vi "HOST_feedbacktest1_AAoptAOD_8-8-23.vi"() -> ()   [LabVIEW 2020]
uses:
  <vilib>/userDefined/Silver/nirio_resource_slv.ctl
  Controls/Clock Select.ctl
  <vilib>/rvi/Analysis/control/PID/Typedef/niFpgaPID_ManualControl.ctl
  <vilib>/rvi/Analysis/control/PID/Typedef/niFpgaPID_PIDGains.ctl
  <vilib>/rvi/Analysis/control/PID/Typedef/niFpgaPID_OutputRange.ctl
  <vilib>/rvi/Analysis/control/PID/Typedef/niFpgaPID_SetpointWeightings.ctl
  <vilib>/rvi/Analysis/host/Butterworth/config/Butterworth Filter Order.ctl
  <vilib>/rvi/Analysis/host/Butterworth/config/Butterworth Filter Type.ctl
  <vilib>/FPGAPlugInAG/PXIe-7972R/niLvFpga_Open_PXIe-7972R.vi
  <vilib>/rvi/interface/common/dynamic/niFpgaDynamicAddResources.vi
  <vilib>/rvi/interface/common/niFpgaWaitOnOcc.vi
  <vilib>/Utility/error.llb/Error Cluster From Error Code.vi
  <vilib>/rvi/Analysis/host/Butterworth/config/BwScaledCoefficients.vi
  <vilib>/Utility/file.llb/Write Delimited Spreadsheet (string).vi
  <vilib>/rvi/errors/niLvFpgaAdjustHostInterfaceError.vi
  <instrlib>/_niInstr/Streaming/v1/Host/Public/Start Finite Stream.vi
  <instrlib>/_niInstr/Streaming/v1/Host/Public/Wait for Stream.vi
  <instrlib>/_niInstr/Streaming/v1/Host/Public/Start Continuous Stream.vi
  <vilib>/FPGAPlugInAG/Dynamic/niLvFpga_Close_Dynamic.vi
  <vilib>/rvi/interface/nirviOpenFPGA/nirviOpenFPGA.xnode
  FPGA Bitfiles/rfsignal_FPGATarget_feedbacktest1AAo_8pa4StVbrw0.lvbitx
  <vilib>/rvi/interface/nirviMethod/nirviMethod.xnode
  <vilib>/rvi/Analysis/host/Butterworth/XNode/ButterworthCoefficients.xnode
  <vilib>/rvi/interface/nirviReadWriteControl/nirviReadWriteControl.xnode
  <vilib>/rvi/interface/nirviCloseFPGA/nirviCloseFPGA.xnode
  <vilib>/rvi/errors/niLvFpgaMergeErrorWithErrorCode.vi
  <instrlib>/_niInstr/Streaming/v1/Host/niInstr Streaming v1 Host.lvlib
  <vilib>/rvi/interface/Simulation/niFpgaSimulationCallBeginRW.vi
  NiFpgaLv.dll
  <vilib>/rvi/Analysis/host/Public/NI_FpgaMspHost.lvlib
  <vilib>/FPGAPlugInAG/Dynamic/niLvFpga_ConfigureFifo_Dynamic.vi
  <vilib>/FPGAPlugInAG/Dynamic/niLvFpga_StartFifo_Dynamic.vi
  <vilib>/FPGAPlugInAG/Dynamic/niLvFpga_WriteFifo_Dynamic.vi
panel:
  in  "hp freq X 1":dbl=1300.0
  in  "lp freq X 1":dbl=1300.0
  in  "Setpoint Y 2":i16
  in  "Lower lim Y 2":fxp<+/-,16,16>=-300.0
  in  "Upper lim Y 2":fxp<+/-,16,16>=300.0
  in  "D (Y)2":fxp<+/-,16,16>
  in  "I (X)":fxp<+/-,16,16>
  in  "P (X)":fxp<+/-,16,16>
  in  "setpoint weighting 2":T1={"proportional weighting (1)"=1.0, "derivative weighting (0)"=0.0} {"derivative weighting (0)" min=0 max=1; "proportional weighting (1)" min=0 max=1}
  in  "output range 2":T2={"output high (Inf)"=inf, "output low (-Inf)"=-inf}
  in  "gains 2":T3 {"filter coefficient" min=0 max=1; "proportional gain" step=0.125}
  in  "manual control 2":T4
  in  "channel (0) 2":u8
  in  "reset? (F) 2":bool
  in  "Direction switch":bool
  in  "Step gain values":dbl
  in  "?":bool
  in  "% of max CH 1":dbl=85.0
  in  "% of max CH 0":dbl=85.0
  in  "setpoint weighting":T1={"proportional weighting (1)"=1.0, "derivative weighting (0)"=0.0} {"derivative weighting (0)" min=0 max=1; "proportional weighting (1)" min=0 max=1}
  in  "output range":T2={"output high (Inf)"=inf, "output low (-Inf)"=-inf}
  in  "gains":T3 {"filter coefficient" min=0 max=1; "proportional gain" step=0.125}
  in  "manual control":T4
  in  "channel (0)":u8
  in  "reset? (F)":bool
  in  "PID selector":bool
  in  "write time ch0":bool
  in  "Record time for power sweep CH0":bool
  in  "Record time for power sweep CH1":bool
  in  "write time ch1":bool
  in  "save path for power calibration (dialog if empty)":path
  out "time check":u16=16
  in  "Cycles per step":u16=30
  in  "Gain Scan Endpoint (CH1)":dbl[](array[numeric])=[100.0, 100.0, 100.0, 100.0, 100.0, 100.0, 100.0, 100.0, 100.0, 100.0, 100.0, 100.0, 100.0, 100.0, 100.0, 100.0, 100.0, 100.0, 100.0, 100.0, 100.0, 100.0, 100.0, 100.0, 100.0, 100.0, 100.0, 100.0, 100.0, 100.0, 100.0, 100.0, 100.0, 100.0, 100.0, 100.0]
  in  "Gain Scan Endpoint (CH0)":dbl[](array[numeric])=[100.0, 100.0, 100.0, 100.0, 100.0, 100.0, 100.0, 100.0, 100.0, 100.0, 100.0, 100.0, 100.0, 100.0, 100.0, 100.0, 100.0, 100.0, 100.0, 100.0, 100.0, 100.0, 100.0, 100.0, 100.0, 100.0, 100.0, 100.0, 100.0, 100.0, 100.0, 100.0, 100.0, 100.0, 100.0, 100.0]
  in  "Scan End Setpoint (CH1)":dbl[](array[numeric])=[23.0, 24.0, 25.0, 26.0, 27.0, 28.0, 23.0, 24.0, 25.0, 26.0, 27.0, 28.0, 23.0, 24.0, 25.0, 26.0, 27.0, 28.0, 23.0, 24.0, 25.0, 26.0, 27.0, 28.0, 23.0, 24.0, 25.0, 26.0, 27.0, 28.0, 23.0, 24.0, 25.0, 26.0, 27.0, 28.0] format="%#_10f"
  in  "Scan CH1":bool
  in  "Scan CH0":bool
  in  "Fq Scan Endpoint (CH0)":dbl[](array[numeric])=[23.0, 23.0, 23.0, 23.0, 23.0, 23.0, 24.0, 24.0, 24.0, 24.0, 24.0, 24.0, 25.0, 25.0, 25.0, 25.0, 25.0, 25.0, 26.0, 26.0, 26.0, 26.0, 26.0, 26.0, 27.0, 27.0, 27.0, 27.0, 27.0, 27.0, 28.0, 28.0, 28.0, 28.0, 28.0, 28.0] format="%#_10f"
  in  "LP FF":dbl=5000.0 format="%#_13g"
  in  "Refresh Integral":bool
  in  "Setpoint Y 1":i16
  in  "Lower lim Y 1":fxp<+/-,16,16>=-300.0
  in  "Upper lim Y 1":fxp<+/-,16,16>=300.0
  in  "hp freq Y 1":dbl=1300.0
  in  "lp freq Y 1":dbl=1300.0
  in  "Scaling (Y) 1":fxp<+,16,4>=1.0
  in  "D (Y) 1":fxp<+/-,16,16>
  in  "I (Y) 1":fxp<+/-,16,16>
  in  "P (Y) 1":fxp<+/-,16,16>
  in  "Amp mod on/off":bool[](array[boolean])=[FALSE, FALSE, FALSE, FALSE, FALSE, FALSE, FALSE, FALSE, FALSE]
  in  "Mod Amp (%)":fxp<+,16,1>[](array[numeric])=[1.0, 1.0, 1.0, 1.0, 1.0, 1.0, 1.0, 1.0, 1.0]
  in  "Mod Fq (Hz) 3":dbl[](array[numeric])=[1.0, 1.0, 1.0, 1.0, 1.0, 1.0, 1.0, 1.0, 1.0] format="%#5.5f"
  in  "Wave 2 mod on/off":bool[](array[boolean])=[FALSE, FALSE, FALSE, FALSE, FALSE, FALSE, FALSE, FALSE, FALSE]
  in  "Mod strength (Hz) 2":dbl[](array[numeric])=[100000.0, 100000.0, 100000.0, 100000.0, 100000.0, 100000.0, 100000.0, 100000.0, 100000.0] format="%#_6p"
  in  "Mod Fq (Hz) 2":dbl[](array[numeric])=[1.0, 1.0, 1.0, 1.0, 1.0, 1.0, 1.0, 1.0, 1.0] format="%#5.5f"
  in  "Wave 1 mod on/off":bool[](array[boolean])=[FALSE, FALSE, FALSE, FALSE, FALSE, FALSE, FALSE, FALSE, FALSE]
  in  "Mod strength (Hz)":dbl[](array[numeric])=[100000.0, 100000.0, 100000.0, 100000.0, 100000.0, 100000.0, 100000.0, 100000.0, 100000.0] format="%#_6p"
  in  "Mod Time (Hz)":dbl[](array[numeric])=[1.0, 1.0, 1.0, 1.0, 1.0, 1.0, 1.0, 1.0, 1.0] format="%#5.5p"
  in  "Gain Scan Step Size % (CH1)":dbl=1.0
  in  "Gain Scan Step Size % (CH0)":dbl=1.0
  in  "Fq Scan Step Size MHz (CH1)":dbl=0.1
  in  "Fq Scan Step Size MHz (CH0)":dbl=0.1
  in  "Input pass through\nmode":enum16{"Wire", "Accum", "Accum-edge"}(ring)
  in  "# of beams":i8=36
  in  "Wave Reader CH 1 (MHz)":dbl[](array[numeric])=[23.0, 24.0, 25.0, 26.0, 27.0, 28.0, 23.0, 24.0, 25.0, 26.0, 27.0, 28.0, 23.0, 24.0, 25.0, 26.0, 27.0, 28.0, 23.0, 24.0, 25.0, 26.0, 27.0, 28.0, 23.0, 24.0, 25.0, 26.0, 27.0, 28.0, 23.0, 24.0, 25.0, 26.0, 27.0, 28.0] format="%#_15f"
  in  "Gain CH 1 (%)":dbl[](array[numeric])=[100.0, 100.0, 100.0, 100.0, 100.0, 100.0, 100.0, 100.0, 100.0, 100.0, 100.0, 100.0, 100.0, 100.0, 100.0, 100.0, 100.0, 100.0, 100.0, 100.0, 100.0, 100.0, 100.0, 100.0, 100.0, 100.0, 100.0, 100.0, 100.0, 100.0, 100.0, 100.0, 100.0, 100.0, 100.0, 100.0]
  in  "Remove transition edges":i32=5
  in  "Time per beam in us":i32=20
  in  "stop":bool
  in  "Gain CH 0 (%)":dbl[](array[numeric])=[100.0, 100.0, 100.0, 100.0, 100.0, 100.0, 100.0, 100.0, 100.0, 100.0, 100.0, 100.0, 100.0, 100.0, 100.0, 100.0, 100.0, 100.0, 100.0, 100.0, 100.0, 100.0, 100.0, 100.0, 100.0, 100.0, 100.0, 100.0, 100.0, 100.0, 100.0, 100.0, 100.0, 100.0, 100.0, 100.0]
  in  "Wave Reader CH 0 (MHz)":dbl[](array[numeric])=[23.0, 23.0, 23.0, 23.0, 23.0, 23.0, 24.0, 24.0, 24.0, 24.0, 24.0, 24.0, 25.0, 25.0, 25.0, 25.0, 25.0, 25.0, 26.0, 26.0, 26.0, 26.0, 26.0, 26.0, 27.0, 27.0, 27.0, 27.0, 27.0, 27.0, 28.0, 28.0, 28.0, 28.0, 28.0, 28.0] format="%#_13f"
  in  "Magnitude Initialization Vpp":dbl[](array[numeric])=[1.0, 1.0] format="%0.2p"
  in  "Frequencies (Hz)":dbl[](array[numeric])=[10000.0, 10000.0] format="%5.0p"
  in  "Signal Type":T5(ring)
  in  "Sampling Info":cluster{"Fs":dbl, "#s":dbl}={"Fs"=163840000.0, "#s"=65536.0} {"Fs" format="%#_5p"}
  out "Error Out":errorcluster
  in  "Update Waveform":bool
  in  "Clock Select":T6 items=["Internal Clock", "Internal Clock w/ Ref via CLK/REF IN", "Internal Clock w/ Ref via Sync Clock", "External Clock via CLK/REF IN"]
  in  "Rate of External Sample Clock (MHz)":u16=100 min=60 max=100 step=1
  in  "RIO Resource":T7="RIO0"
  # "General Feedback Settings"
  # "Time cycle loop processing"
  # "Shared Feedback Controls"
  # "Don't change"
  # "Waveform Initialization"
  # "Beam 1 Feedback Parameters"
  # "Modulation disabled for now while testing FPGA code, too high compiling time for quick turn around"
  # "Controls the Output of the FPGA\nEach row corresponds to one beam created by the AOD\nCH 0 is Output 0 on the FPGA card and controls the () direction on the AOD; CH 1 is Output 1 on the FPGA card and controls the () direction on the AOD\n\nThe  set frequency is the output of the FPGA, this is then mixed with a 50MHz LO to be in the AOD's bandwidth of 75 +- 15MHz\n\nThe gain is the percentage of the 1Vpp initialized voltage to output. It is in percentage and goes from 0 - 100\n\nIt will play the first n rows of tones, \nwhere n is the \"# of beams\" value."
  # "DO NOT CHANGE"
  # "These allow you to smoothly ramp between frequencies or gain settings for each individual beam.\nThe channels scan independently, but it will simultaneously ramp every fq/gain in the channel to their desired point.\nThey should update to match the main control setting when scanning is not enabled."
  # "AI 0 Controls Labview Sample PID"
  # "AI 1 Controls Labview Sample PID"
  # "Ch 0 Wave Sin Modulation"
  # "Ch 1 Wave Sin Modulation"
  # "Amplitude Sin Modulation"
  # "Do not change these values while waiting for scan"
  # "Main control for the tones played on FPGA analog out 0\nSets the base, static frequency to play"
  # "Main control for the tones played on FPGA analog out 1\nSets the base, static frequency to play"
  # "Ch 0 Output Waveforms"
  # "Ch 1 Output Waveforms"
  # "Limits go as fractions of maxI16 (for testing purposes)\n1 means I16 positively saturated (dac output rails positive)\n-1 means I16 negatively saturated (dac output rails negative)\ndefined in PID subvi on the FPGA"
  # "Ch0"
  # "Ch1"
  # "Modulates the output frequencies of CH 0 in a sine wave pattern\n\nMod time: Sets how fast the modulation goes\n     (e.g. 1 Hz means it will go through a full cycle in 1 second)\n\nMod strength: Sets the amplitude of the modulation\n     (e.g. 100kHz means that the frequency will go between \n      set frequency + 100kHz and set frequency - 100kHz)"
  # "Modulates the output frequencies of CH 1 in a sine wave pattern\n\nMod time: Sets how fast the modulation goes\n     (e.g. 1 Hz means it will go through a full cycle in 1 second)\n\nMod strength: Sets the amplitude of the modulation\n     (e.g. 100kHz means that the frequency will go between \n      set frequency + 100kHz and set frequency - 100kHz)"
  # "Modulates the output amplitude of CH 0 in a sine wave pattern\n\nMod time: Sets how fast the modulation goes\n     (e.g. 1 Hz means it will go through a full cycle in 1 second)\n\nMod strength: Sets the amplitude of the modulation\n     (e.g. 5% means that the amplitude will go between \n      set amp + 5%  and set amp  - 5%)"
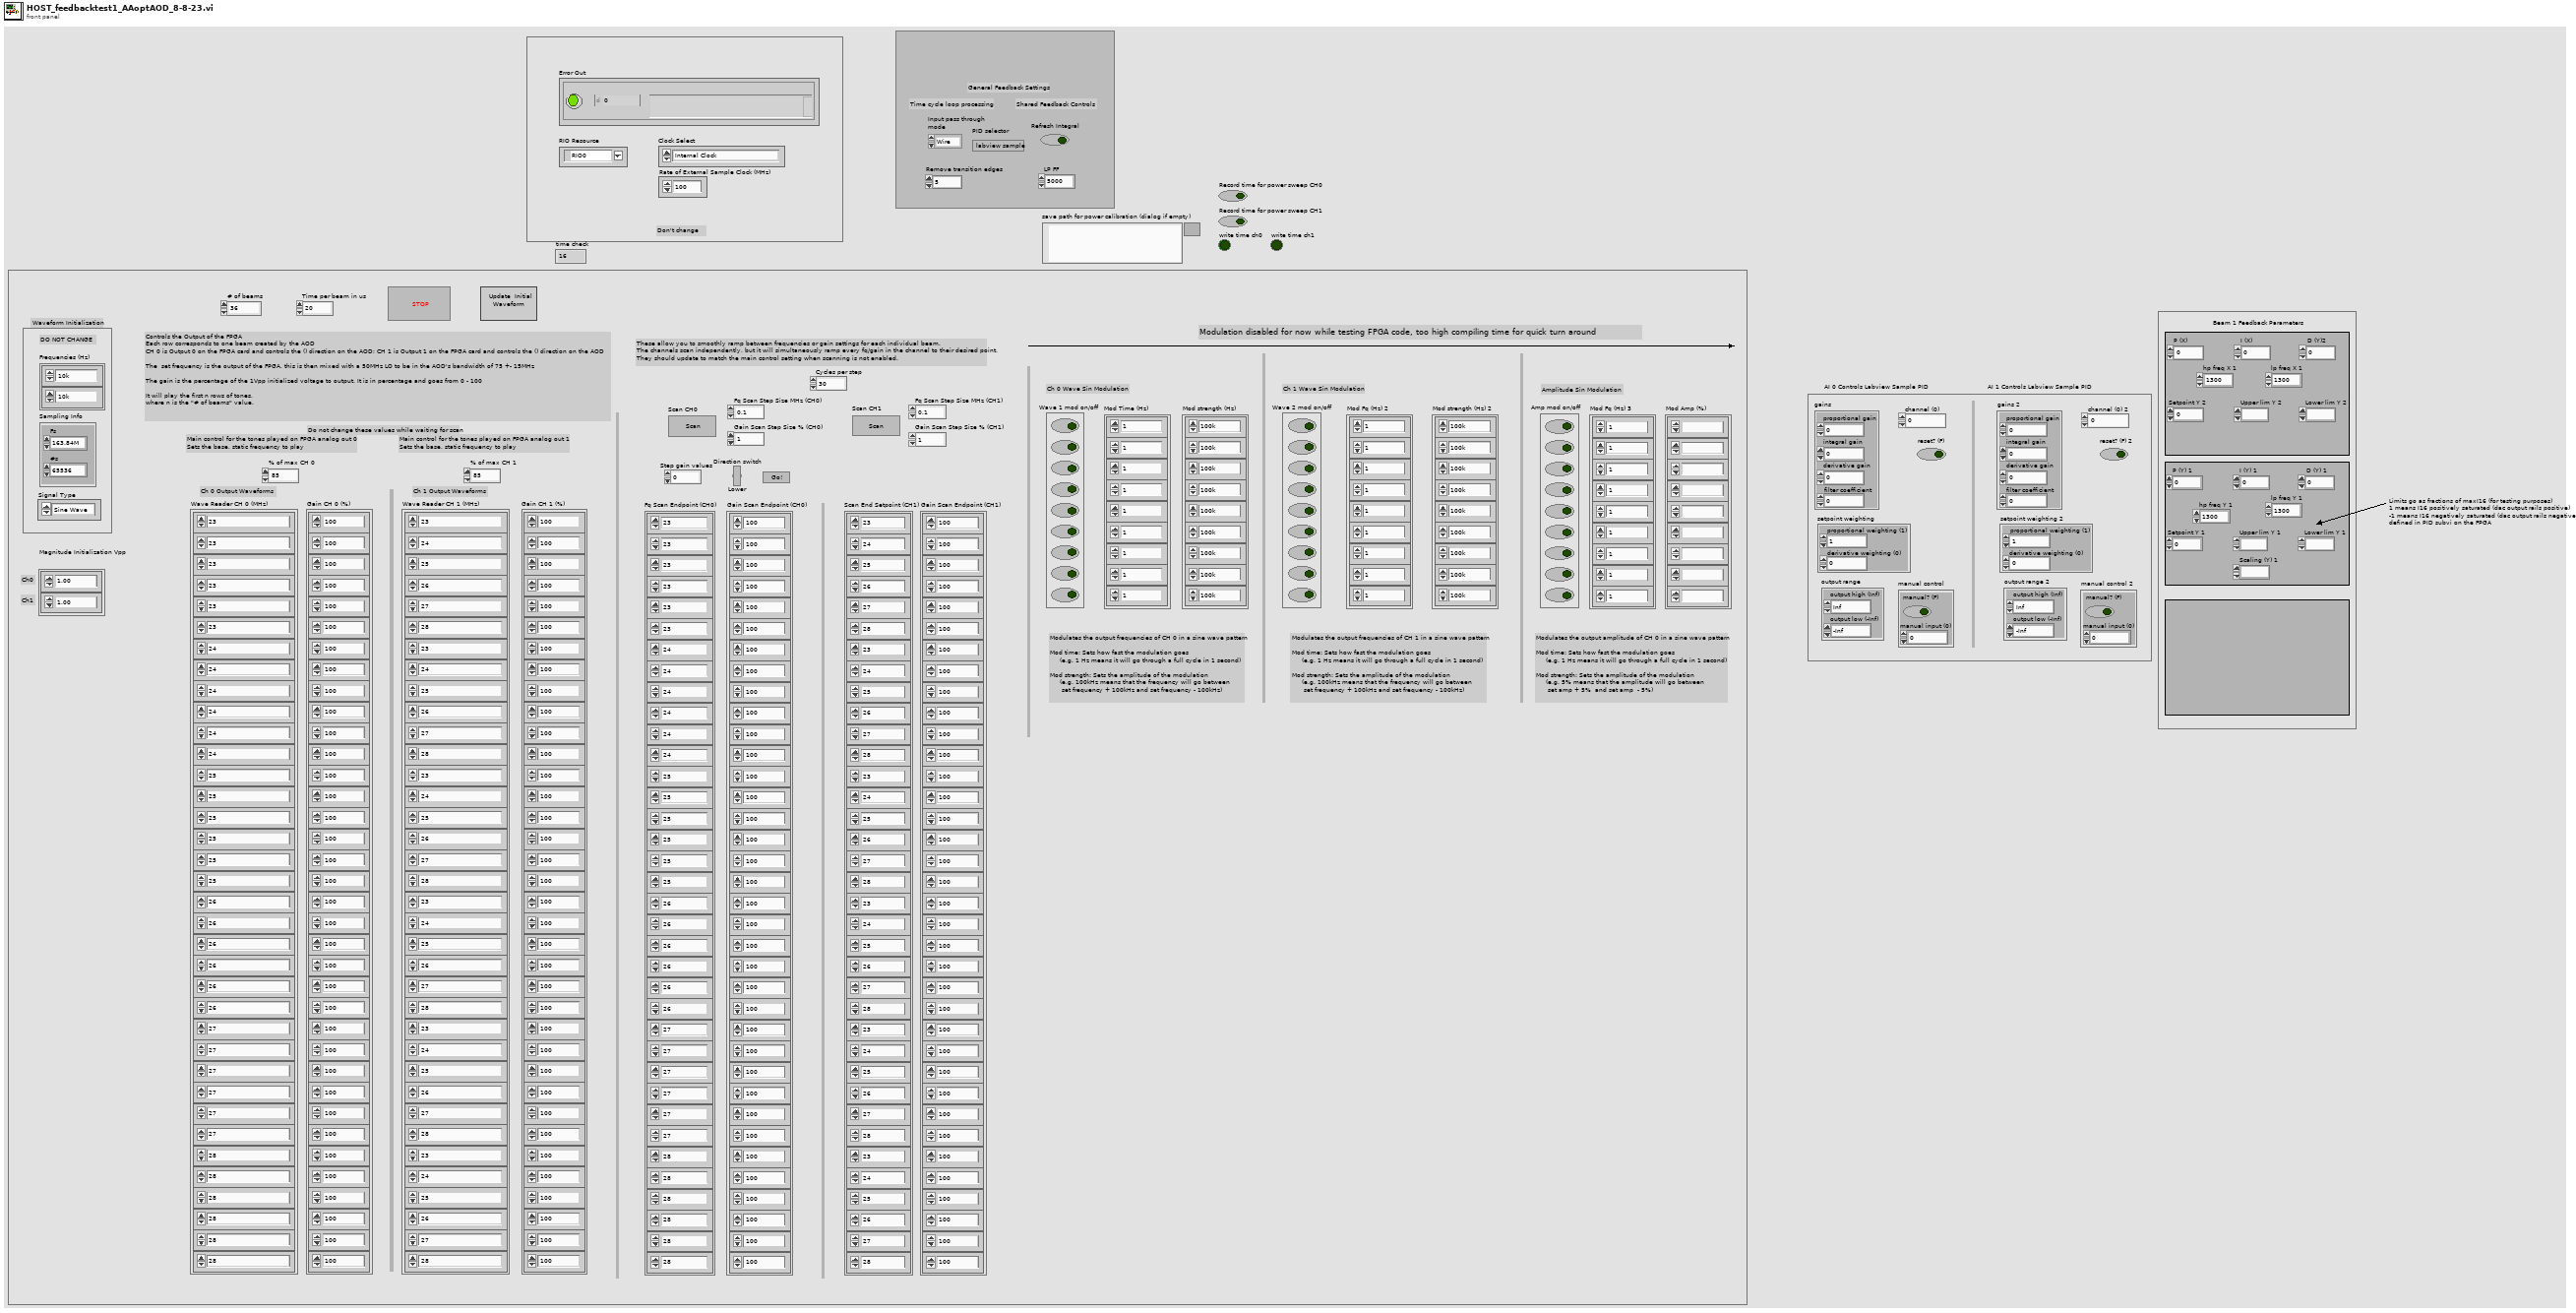
[diagram p1: front panel]
types:
  T1 = typedef "niFpgaPID_SetpointWeightings.ctl" = cluster{"proportional weighting (1)":sgl, "derivative weighting (0)":sgl}
  T2 = typedef "niFpgaPID_OutputRange.ctl" = cluster{"output high (Inf)":sgl, "output low (-Inf)":sgl}
  T3 = typedef "niFpgaPID_PIDGains.ctl" = cluster{"proportional gain":sgl, "integral gain":sgl, "derivative gain":sgl, "filter coefficient":sgl}
  T4 = typedef "niFpgaPID_ManualControl.ctl" = cluster{"manual? (F)":bool, "manual input (0)":sgl}
  T5 = enum16{"Sine Wave", "Triangle Wave", "Square Wave", "Sawtooth Wave"}
  T6 = typedef "Clock Select.ctl" = u16
  T7 = typedef "nirio_resource_slv.ctl" = tag
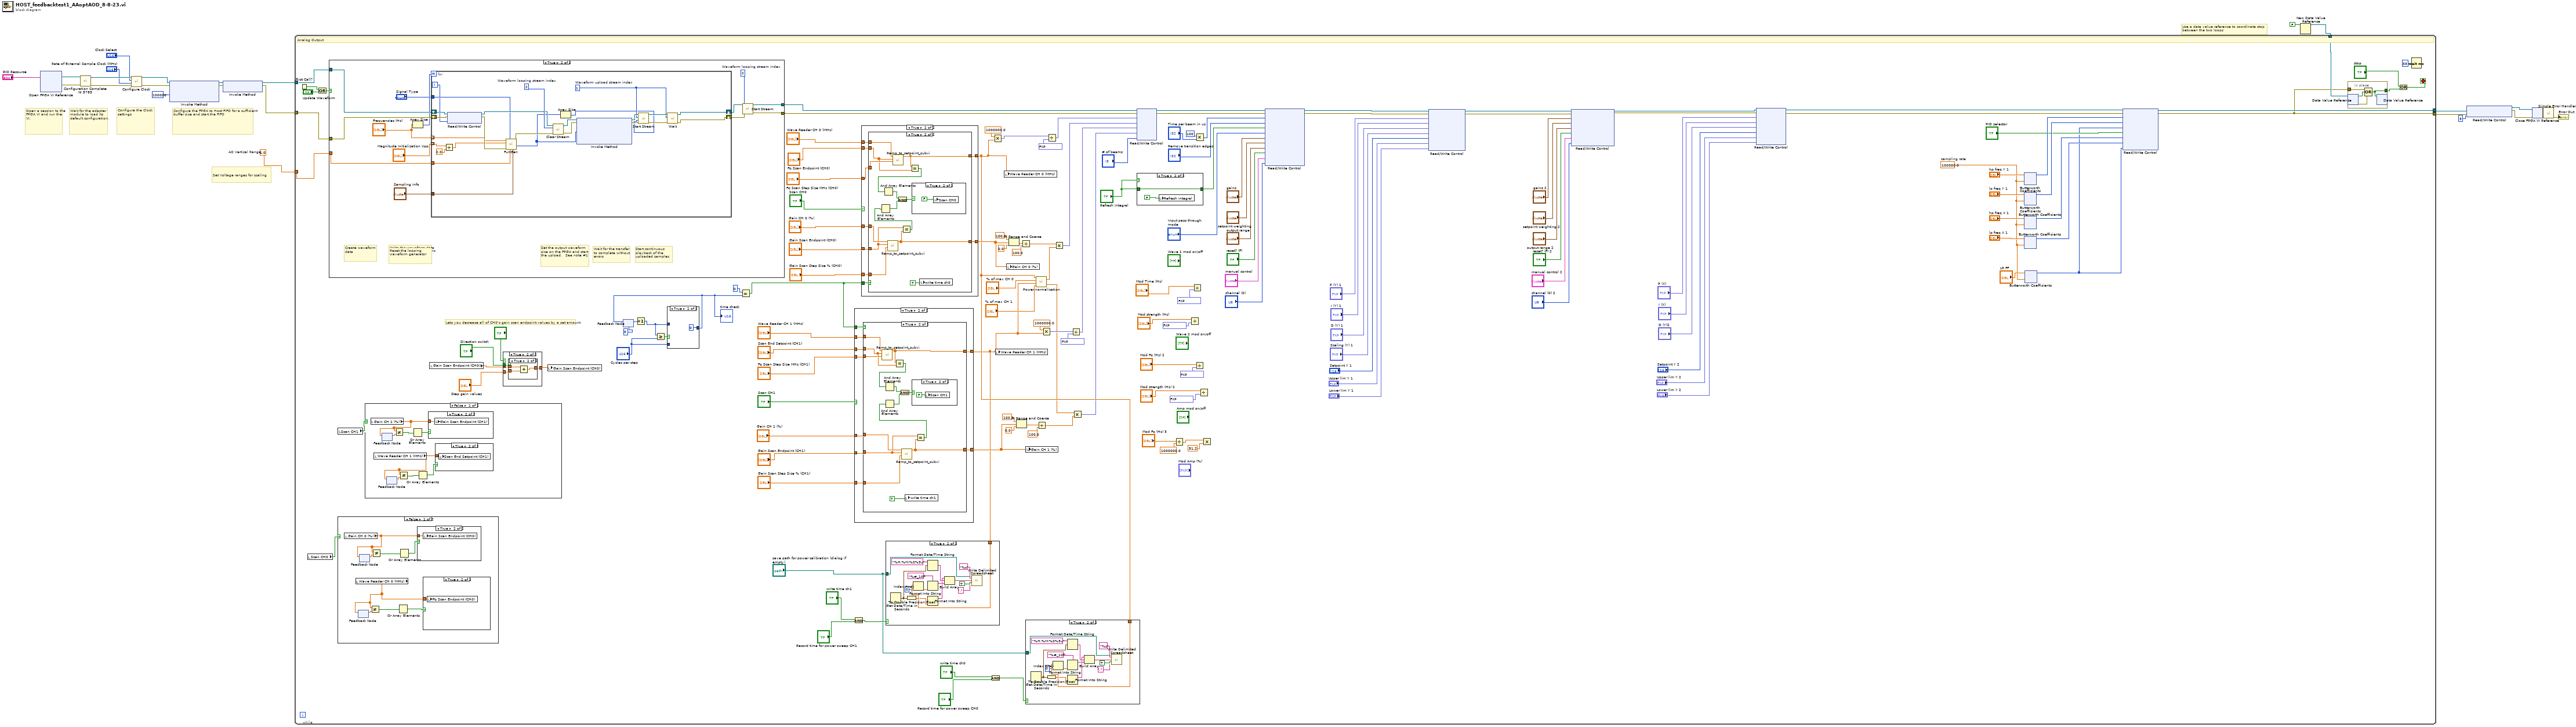
[diagram p0: block diagram]
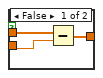
[diagram p3: hidden frame]
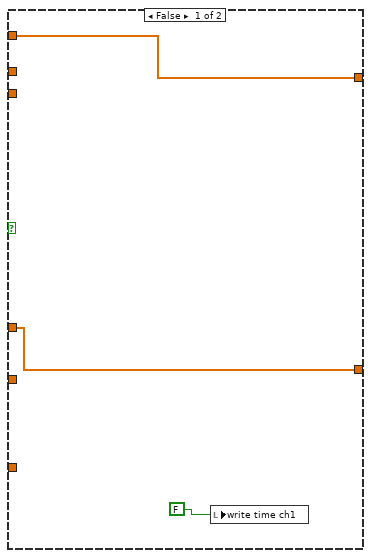
[diagram p6: hidden frame]
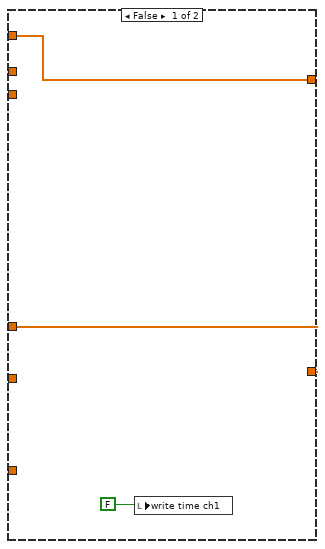
[diagram p7: hidden frame]
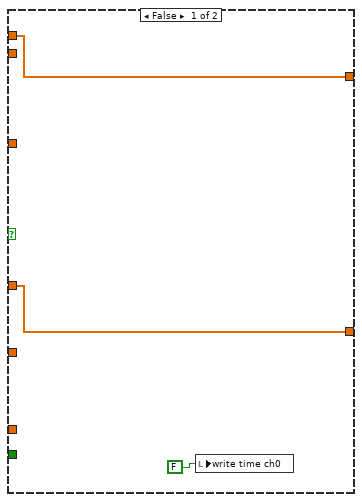
[diagram p9: hidden frame]
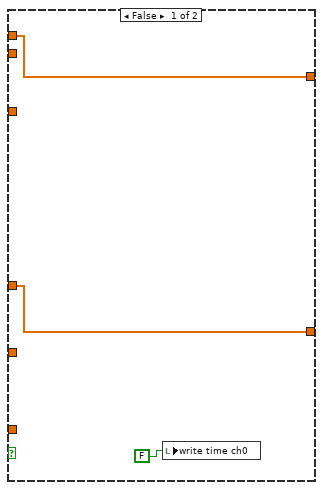
[diagram p10: hidden frame]
diagram:
  w12 = 1.0  # AO Vertical Range
  # "Use a data value reference to coordinate stop between the two loops"
  # "Set Voltage ranges for scaling"
  # "Configure the Clock settings"
  # "Configure the FPGA to Host FIFO for a sufficient buffer size and start the FIFO"
  # "Wait for the adapter module to load its default configuration."
  # "Open a session to the FPGA VI and run the VI."
  n1 = xnode "Open FPGA VI Reference"("resource name"="RIO Resource") -> ("FPGA VI Reference Out"=w10:refnum<k20>, "error out"=w9:errorcluster)  [unwired: 1 in]
  n2 = call "Configuration Complete NI 5783.vi"("error in"=w9, "FPGA VI Reference In"=w10) -> ("error out"=w20:errorcluster, "FPGA VI Reference Out"=w21:refnum<k20>)  [unwired: 7 in, 1 out]
  n3 = call "Configure Clock.vi"("error in (no error)"=w20, "Rate of External Sample Clock (MHz)"="Rate of External Sample Clock (MHz)", "Clock Select"="Clock Select", "FPGA VI Reference In"=w21) -> ("error out"=w18:errorcluster, "FPGA VI Reference Out"=w19:refnum<k20>)  [unwired: 3 in, 3 out]
  n4 = xnode "Invoke Method"("FPGA VI Reference In"=w19, "error in"=w18, "Requested Depth"=u32 100000) -> ("FPGA VI Reference Out"=w24:refnum<k20>, "error out"=w23:errorcluster)  [unwired: 1 out]
  n5 = xnode "Invoke Method"("FPGA VI Reference In"=w24, "error in"=w23) -> ("FPGA VI Reference Out"=w3:refnum<k20>, "error out"=w2:errorcluster)
  n6 = New Data Value Reference(data value=FALSE ("Stopped")) -> (data value reference=w1:refnum<data-value>)  [unwired: 1 in, 1 out]
  n7 = while {
    tunnel: w2 -> [w164]
    tunnel: [w119] -> w8
    tunnel: w3 -> [w170]
    tunnel: [w122] -> w7
    tunnel: w1 -> [w165]
    tunnel: w12 -> [w163]
    stop <- w160 stop-if-true
    w26 = 100000.0  # sampling rate
    # "Lets you decrease all of CH0's gain scan endpoint values by a set amount"
    # "Analog Output"
    n8 = First Call?() -> (First Call?: T/F=w166:bool)
    n9 = local read "Scan CH0"() -> (w93:bool)
    n10 = Or(x=w166, y="Update Waveform") -> (x .or. y?=w167:bool)
    n11 = case shown="True" w167 {
      tunnel: [w337 w350] -> w162
      tunnel: [w336 w349] -> w161
      tunnel: w170 -> [w337 w347]
      tunnel: w164 -> [w336 w346]
      tunnel: w163 -> [_ w348]
      frame False {
      }
      frame True {
        w345 = 2  # Waveform looping stream index
        # "Loop over the waveforms to combine"
        # "Reset the looping waveform generator"
        # "Start continuous playback of the uploaded samples"
        # "Wait for the transfer to complete without errors"
        # "Set the output waveform size on the FPGA and start the upload.   See note #1"
        # "Write the waveform data to the FPGA for generation"
        # "Create waveform data"
        n12 = Array Size(array="Frequencies (Hz)") -> (size(s)=w340:i32)
        n13 = for {
          N: w340 -> [_]
          tunnel: w348 -> [w365]
          shift-right: [w359] -> w344
          shift-left: w347 -> [w364]
          shift-right: [w358] -> w343
          shift-left: w346 -> [w362]
          tunnel: "Frequencies (Hz)" -> [w357] mode=indexing
          tunnel: "Magnitude Initialization Vpp" -> [w353] mode=indexing
          tunnel: "Sampling Info" -> [w356]
          tunnel: "Signal Type" -> [w355]
          i -> [w354]
          w366 = 2  # Waveform looping stream index
          w371 = 1  # Waveform upload stream index
          n14 = Divide(x=w353, y=2.0) -> (x/y=w352:dbl)
          n15 = xnode "Read/Write Control"("FPGA VI Reference In"=w364, "error in"=w362, "Upload selector"=w354) -> ("FPGA VI Reference Out"=w363:refnum<k20>, "error out"=w361:errorcluster)
          n16 = call "FunGen.vi"("sampling info"=w356, "range (Vpp)"=w365, "signal type"=w355, "error in (no error)"=w361, "amplitude"=w352, "frequency"=w357) -> ("error out"=w367:errorcluster, "Waveform Data"=w360:i16[])  [unwired: 2 in, 2 out]
          n17 = call <instrlib>:"Clear Stream.vi"("error in (no error)"=w367, "stream index"=w366, "refnum in"=w363) -> ("error out"=w369:errorcluster, "refnum out"=w370:refnum<k20>)  [unwired: 7 in]
          n18 = Array Size(array=w360) -> (size(s)=w368:i32)
          n19 = xnode "Invoke Method"("FPGA VI Reference In"=w370, "error in"=w369, "Data"=w360) -> ("FPGA VI Reference Out"=w375:refnum<k20>, "error out"=w374:errorcluster)  [unwired: 1 in, 1 out]
          n20 = call-poly <instrlib>:"Start Stream.vi"("error in (no error)"=w374, "num samples"=w368, "stream index"=w371, "refnum in"=w375) -> ("error out"=w372:errorcluster, "refnum out"=w373:refnum<k20>)  [unwired: 6 in]
          n21 = call-poly <instrlib>:"Wait.vi"("error in (no error)"=w372, "stream index"=w371, "refnum in"=w373) -> ("error out"=w358:errorcluster, "refnum out"=w359:refnum<k20>)  [unwired: 5 in, 2 out]
        }
        n22 = call-poly <instrlib>:"Start Stream.vi"("error in (no error)"=w343, "stream index"=w345, "refnum in"=w344) -> ("error out"=w349:errorcluster, "refnum out"=w350:refnum<k20>)  [unwired: 7 in]
      }
    }
    n23 = local read "Scan CH1"() -> (w94:bool)
    n24 = case shown="False" w93 {
      frame False {
        n25 = local read "Gain CH 0 (%)"() -> (w288:dbl[])
        n26 = local read "Wave Reader CH 0 (MHz)"() -> (w295:dbl[])
        n27 = feedback-in #1(w295) -> ()
        n28 = feedback #1() -> (w294:dbl[])  [unwired: 1 in]
        n29 = feedback #2() -> (w291:dbl[])  [unwired: 1 in]
        n30 = feedback-in #2(w288) -> ()
        n31 = Not Equal?(x=w295, y=w294) -> (x != y?=w293:bool[])
        n32 = Not Equal?(x=w288, y=w291) -> (x != y?=w290:bool[])
        n33 = Or Array Elements(Boolean array=w293) -> (logical OR=w292:bool)
        n34 = Or Array Elements(Boolean array=w290) -> (logical OR=w289:bool)
        n35 = case shown="True" w289 {
          tunnel: w288 -> [_ w296]
          frame False {
          }
          frame True {
            n36 = local write "Gain Scan Endpoint (CH0)"(w296) -> ()
          }
        }
        n37 = case shown="True" w292 {
          tunnel: w295 -> [_ w297]
          frame False {
          }
          frame True {
            n38 = local write "Fq Scan Endpoint (CH0)"(w297) -> ()
          }
        }
      }
      frame True {
      }
    }
    n39 = case shown="False" w94 {
      frame False {
        n40 = local read "Gain CH 1 (%)"() -> (w298:dbl[])
        n41 = local read "Wave Reader CH 1 (MHz)"() -> (w302:dbl[])
        n42 = feedback #3() -> (w301:dbl[])  [unwired: 1 in]
        n43 = feedback-in #3(w298) -> ()
        n44 = feedback #4() -> (w305:dbl[])  [unwired: 1 in]
        n45 = feedback-in #4(w302) -> ()
        n46 = Not Equal?(x=w298, y=w301) -> (x != y?=w300:bool[])
        n47 = Not Equal?(x=w302, y=w305) -> (x != y?=w304:bool[])
        n48 = Or Array Elements(Boolean array=w300) -> (logical OR=w299:bool)
        n49 = Or Array Elements(Boolean array=w304) -> (logical OR=w303:bool)
        n50 = case shown="True" w299 {
          tunnel: w298 -> [_ w306]
          frame False {
          }
          frame True {
            n51 = local write "Gain Scan Endpoint (CH1)"(w306) -> ()
          }
        }
        n52 = case shown="True" w303 {
          tunnel: w302 -> [_ w307]
          frame False {
          }
          frame True {
            n53 = local write "Scan End Setpoint (CH1)"(w307) -> ()
          }
        }
      }
      frame True {
      }
    }
    n54 = local read "Gain Scan Endpoint (CH0)"() -> (w50:dbl[])
    n55 = case shown="True" "?" {
      tunnel: w50 -> [w185 w188]
      tunnel: [w185 w189] -> w51
      tunnel: "Step gain values" -> [_ w187]
      tunnel: "Direction switch" -> [_ w186]
      frame False {
      }
      frame True {
        n56 = case shown="True" w186 {
          tunnel: [w192 w194] -> w189
          tunnel: w188 -> [w191 w193]
          tunnel: w187 -> [w190 w195]
          frame False {
            n57 = Subtract(x=w191, y=w190) -> (x-y=w192:dbl[])
          }
          frame True {
            n58 = Add(x=w193, y=w195) -> (x+y=w194:dbl[])
          }
        }
      }
    }
    n59 = local write "Gain Scan Endpoint (CH0)"(w51) -> ()
    n60 = feedback #5(u16 0) -> (w89:u16)
    n61 = Increment(x=w89) -> (x+1=w87:u16)
    n62 = Greater Or Equal?(x=w87, y="Cycles per step") -> (x >= y?=w88:bool)
    n63 = case shown="True" w88 {
      tunnel: w87 -> [w286 _]
      tunnel: "Cycles per step" -> [_ _]
      tunnel: [w286 u16 0] -> w82
      frame False {
      }
      frame True {
      }
    }
    "time check" <- w82
    n64 = feedback-in #5(w82) -> ()
    n65 = Equal?(x=u16 0, y=w82) -> (x = y?=w83:bool)
    n66 = And(x="write time ch1", y="Record time for power sweep CH1") -> (x .and. y?=w81:bool)
    n67 = case shown="True" "Scan CH1" {
      tunnel: "Fq Scan Step Size MHz (CH1)" -> [_ w237]
      tunnel: [w228 w236] -> w59
      tunnel: "Wave Reader CH 1 (MHz)" -> [w228 w235]
      tunnel: "Scan End Setpoint (CH1)" -> [_ w234]
      tunnel: "Gain Scan Step Size % (CH1)" -> [_ w233]
      tunnel: "Gain CH 1 (%)" -> [w227 w232]
      tunnel: "Gain Scan Endpoint (CH1)" -> [_ w231]
      tunnel: [w227 w230] -> w95
      tunnel: w83 -> [_ w229]
      frame False {
        n68 = local write "write time ch1"(FALSE) -> ()
      }
      frame True {
        n69 = case shown="True" w229 {
          tunnel: w235 -> [w240 w254]
          tunnel: w234 -> [_ w252]
          tunnel: w237 -> [_ w253]
          tunnel: [w240 w251] -> w236
          tunnel: w232 -> [w239 w249]
          tunnel: w231 -> [_ w248]
          tunnel: w233 -> [_ w247]
          tunnel: [w239 w242] -> w230
          frame False {
            n70 = local write "write time ch1"(FALSE) -> ()
          }
          frame True {
            n71 = call "Ramp_to_setpoint_subvi.vi"("Numeric"=w253, "Scan to Fq (CH0)"=w252, "Wave Reader CH 0 (Y)"=w254) -> ("Array"=w251:dbl[])  [unwired: 8 in]
            n72 = Equal?(x=w251, y=w252) -> (x = y?=w250:bool[])
            n73 = And Array Elements(Boolean array=w250) -> (logical AND=w244:bool)
            n74 = call "Ramp_to_setpoint_subvi.vi"("Numeric"=w247, "Scan to Fq (CH0)"=w248, "Wave Reader CH 0 (Y)"=w249) -> ("Array"=w242:dbl[])  [unwired: 8 in]
            n75 = local write "write time ch1"(TRUE) -> ()
            n76 = Equal?(x=w248, y=w242) -> (x = y?=w243:bool[])
            n77 = And Array Elements(Boolean array=w243) -> (logical AND=w245:bool)
            n78 = And(x=w244, y=w245) -> (x .and. y?=w246:bool)
            n79 = case shown="True" w246 {
              frame False {
              }
              frame True {
                n80 = local write "Scan CH1"(FALSE) -> ()
              }
            }
          }
        }
      }
    }
    n81 = case shown="True" "Scan CH0" {
      tunnel: "Fq Scan Step Size MHz (CH0)" -> [_ w267]
      tunnel: "Wave Reader CH 0 (MHz)" -> [w258 w266]
      tunnel: "Fq Scan Endpoint (CH0)" -> [_ w265]
      tunnel: [w258 w264] -> w60
      tunnel: "Gain CH 0 (%)" -> [w257 w263]
      tunnel: "Gain Scan Endpoint (CH0)" -> [_ w262]
      tunnel: [w257 w261] -> w103
      tunnel: "Gain Scan Step Size % (CH0)" -> [_ w260]
      tunnel: w83 -> [_ w259]
      frame False {
        n82 = local write "write time ch0"(FALSE) -> ()
      }
      frame True {
        n83 = case shown="True" w259 {
          tunnel: w266 -> [w270 w284]
          tunnel: w265 -> [_ w282]
          tunnel: w267 -> [_ w283]
          tunnel: [w270 w281] -> w264
          tunnel: w263 -> [w269 w279]
          tunnel: w262 -> [_ w276]
          tunnel: w260 -> [_ w278]
          tunnel: [w269 w277] -> w261
          frame False {
            n84 = local write "write time ch0"(FALSE) -> ()
          }
          frame True {
            n85 = call "Ramp_to_setpoint_subvi.vi"("Numeric"=w278, "Scan to Fq (CH0)"=w276, "Wave Reader CH 0 (Y)"=w279) -> ("Array"=w277:dbl[])  [unwired: 8 in]
            n86 = call "Ramp_to_setpoint_subvi.vi"("Numeric"=w283, "Scan to Fq (CH0)"=w282, "Wave Reader CH 0 (Y)"=w284) -> ("Array"=w281:dbl[])  [unwired: 8 in]
            n87 = Equal?(x=w276, y=w277) -> (x = y?=w275:bool[])
            n88 = And Array Elements(Boolean array=w275) -> (logical AND=w272:bool)
            n89 = Equal?(x=w281, y=w282) -> (x = y?=w280:bool[])
            n90 = And Array Elements(Boolean array=w280) -> (logical AND=w273:bool)
            n91 = And(x=w273, y=w272) -> (x .and. y?=w274:bool)
            n92 = case shown="True" w274 {
              frame False {
              }
              frame True {
                n93 = local write "Scan CH0"(FALSE) -> ()
              }
            }
            n94 = local write "write time ch0"(TRUE) -> ()
          }
        }
      }
    }
    n95 = case shown="True" w81 {
      tunnel: w59 -> [_ w218]
      tunnel: "save path for power calibration (dialog if empty)" -> [_ w211]
      frame False {
      }
      frame True {
        n96 = Get Date/Time In Seconds() -> (seconds since 1Jan1904=w214:timestamp)
        n97 = To Double Precision Float(number=w214) -> (double precision float=w213:dbl)
        n98 = Index Array(array=w218, index=0) -> (element=w216:dbl)
        n99 = Format Date/Time String(time format string (%c)="%H:%M:%S%3u", seconds (now)=w214) -> (date/time string=w221:string)  [unwired: 1 in]
        n100 = Format Into String(format string="%#_10f", w216) -> (resulting string=w220:string)  [unwired: 2 in, 1 out]
        n101 = Format Into String(w213) -> (resulting string=w212:string)  [unwired: 3 in, 1 out]
        n102 = Build Array(w212, w221, w220) -> (w215:string[])
        n103 = call-poly <vilib>:"Write Delimited Spreadsheet.vi"("file path (dialog if empty)"=w211, "format (%s)"="%s" ("format (%.3f)"), "1D data"=w215, "append to file? (new file:F)"=TRUE, "delimiter (\\t)"="," ("delimiter (\\t)")) -> ()  [unwired: 9 in, 2 out]
      }
    }
    n104 = And(x="write time ch0", y="Record time for power sweep CH0") -> (x .and. y?=w77:bool)
    n105 = Multiply(x=1000000.0, y=w60) -> (x*y=w115:fxp<+/-,64,32>[])
    n106 = local write "Wave Reader CH 1 (MHz)"(w59) -> ()
    n107 = local write "Wave Reader CH 0 (MHz)"(w60) -> ()
    n108 = local write "Gain CH 0 (%)"(w103) -> ()
    n109 = In Range and Coerce(upper limit=100.0, x=w103, lower limit=0.0) -> (coerced(x)=w106:dbl[])  [unwired: 1 out]
    n110 = In Range and Coerce(upper limit=100.0, x=w95, lower limit=0.0) -> (coerced(x)=w101:dbl[])  [unwired: 1 out]
    n111 = Divide(x=w106, y=100.0) -> (x/y=w64:dbl[])
    n112 = local write "Gain CH 1 (%)"(w95) -> ()
    n113 = case shown="True" w77 {
      tunnel: w60 -> [_ w203]
      tunnel: "save path for power calibration (dialog if empty)" -> [_ w196]
      frame False {
      }
      frame True {
        n114 = Get Date/Time In Seconds() -> (seconds since 1Jan1904=w199:timestamp)
        n115 = To Double Precision Float(number=w199) -> (double precision float=w198:dbl)
        n116 = Index Array(array=w203, index=0) -> (element=w201:dbl)
        n117 = Format Date/Time String(time format string (%c)="%H:%M:%S%3u", seconds (now)=w199) -> (date/time string=w206:string)  [unwired: 1 in]
        n118 = Format Into String(format string="%#_10f", w201) -> (resulting string=w205:string)  [unwired: 2 in, 1 out]
        n119 = Format Into String(w198) -> (resulting string=w197:string)  [unwired: 3 in, 1 out]
        n120 = Build Array(w197, w206, w205) -> (w200:string[])
        n121 = call-poly <vilib>:"Write Delimited Spreadsheet.vi"("file path (dialog if empty)"=w196, "format (%s)"="%s" ("format (%.3f)"), "1D data"=w200, "append to file? (new file:F)"=TRUE, "delimiter (\\t)"="," ("delimiter (\\t)")) -> ()  [unwired: 9 in, 2 out]
      }
    }
    n122 = call "Power normalization.vi"("% of max CH 1"="% of max CH 1", "CH 1 frequency"=w59, "% of max CH 0"="% of max CH 0", "CH 0 frequency"=w60) -> ("Normalized CH1"=w56:dbl[], "Normalized CH 0"=w61:dbl[])
    n123 = Divide(x=w101, y=100.0) -> (x/y=w57:dbl[])
    n124 = Multiply(x=1000000.0, y=w59) -> (x*y=w112:fxp<+/-,64,32>[])
    n125 = Divide(x=w115, y=fxp<+,32,16> 6103.515625) -> (x/y=w74:fxp<+,33,16>[])
    n126 = Multiply(x=w64, y=w61) -> (x*y=w65:fxp<+,32,4>[])
    n127 = Divide(x=w112, y=fxp<+,32,16> 6103.515625) -> (x/y=w73:fxp<+,33,16>[])
    n128 = Multiply(x=w56, y=w57) -> (x*y=w58:fxp<+,32,4>[])
    n129 = case shown="True" "Refresh Integral" {
      tunnel: [w308 w309] -> w117
      tunnel: "Refresh Integral" -> [w308 w309]
      frame False {
      }
      frame True {
        n130 = local write "Refresh Integral"(FALSE) -> ()
      }
    }
    n131 = xnode "Read/Write Control"("FPGA VI Reference In"=w162, "error in"=w161, "Wave 1"=w74, "Amp 1"=w65, "Wave 2"=w73, "Amp 2"=w58, "Size"="# of beams") -> ("FPGA VI Reference Out"=w156:refnum<k20>, "error out"=w155:errorcluster)
    n132 = Divide(x="Mod Fq (Hz) 3", y=1000000.0) -> (x/y=w141:dbl[])
    n133 = Divide(x="Mod strength (Hz)", y=fxp<+,32,16> 6103.515625) -> ()  [unwired: 1 out]
    n134 = Divide(x="Mod Time (Hz)", y=fxp<+,32,16> 6103.515625) -> ()  [unwired: 1 out]
    n135 = Divide(x="Mod Fq (Hz) 2", y=fxp<+,32,16> 6103.515625) -> ()  [unwired: 1 out]
    n136 = Multiply(x=100, y="Time per beam in us") -> (x*y=w152:i32)
    n137 = Divide(x="Mod strength (Hz) 2", y=fxp<+,32,16> 6103.515625) -> ()  [unwired: 1 out]
    n138 = Multiply(x=w141, y=51.2) -> ()  [unwired: 1 out]
    n139 = xnode "Read/Write Control"("FPGA VI Reference In"=w156, "error in"=w155, "Timeshare"=w152, "Edge size"="Remove transition edges", "Integral reset"=w117, "Pass selector"="Input pass through\nmode", "gains"="gains", "setpoint weighting"="setpoint weighting", "output range"="output range", "reset? (F)"="reset? (F)", "manual control"="manual control", "channel (0)"="channel (0)") -> ("FPGA VI Reference Out"=w145:refnum<k20>, "error out"=w144:errorcluster)
    n140 = xnode "Read/Write Control"("FPGA VI Reference In"=w145, "error in"=w144, "Py gain 1"="P (Y) 1", "Iy gain 1"="I (Y) 1", "Dy gain 1"="D (Y) 1", "Feedback scaling"="Scaling (Y) 1", "Y DC offset 1"="Setpoint Y 1", "Y up lim 1"="Upper lim Y 1", "Y low lim 1"="Lower lim Y 1") -> ("FPGA VI Reference Out"=w36:refnum<k20>, "error out"=w31:errorcluster)
    n141 = xnode "Read/Write Control"("FPGA VI Reference In"=w36, "error in"=w31, "gains 2"="gains 2", "setpoint weighting 2"="setpoint weighting 2", "output range 2"="output range 2", "reset? (F) 2"="reset? (F) 2", "manual control 2"="manual control 2", "channel (0) 2"="channel (0) 2") -> ("FPGA VI Reference Out"=w35:refnum<k20>, "error out"=w32:errorcluster)
    n142 = xnode "Read/Write Control"("FPGA VI Reference In"=w35, "error in"=w32, "Px gain 1"="P (X)", "Ix gain 1"="I (X)", "Dx gain 1"="D (Y)2", "X DC offset 1"="Setpoint Y 2", "X up lim 1"="Upper lim Y 2", "X low lim 1"="Lower lim Y 2") -> ("FPGA VI Reference Out"=w34:refnum<k20>, "error out"=w33:errorcluster)
    n143 = xnode "Butterworth Coefficients"("cutoff frequency (Hz)"="hp freq Y 1", "sample rate (S/s)"=w26) -> ("scaled coefficients"=w121:i32[])  [unwired: 1 in, 1 out]
    n144 = xnode "Butterworth Coefficients"("cutoff frequency (Hz)"="lp freq Y 1", "sample rate (S/s)"=w26) -> ("scaled coefficients"=w120:i32[])  [unwired: 1 in, 1 out]
    n145 = xnode "Butterworth Coefficients"("cutoff frequency (Hz)"="hp freq X 1", "sample rate (S/s)"=w26) -> ("scaled coefficients"=w28:i32[])  [unwired: 1 in, 1 out]
    n146 = xnode "Butterworth Coefficients"("cutoff frequency (Hz)"="lp freq X 1", "sample rate (S/s)"=w26) -> ("scaled coefficients"=w27:i32[])  [unwired: 1 in, 1 out]
    n147 = xnode "Butterworth Coefficients"("cutoff frequency (Hz)"="LP FF", "sample rate (S/s)"=w26) -> ("scaled coefficients"=w25:i32[])  [unwired: 1 in, 1 out]
    n148 = xnode "Read/Write Control"("FPGA VI Reference In"=w34, "error in"=w33, "Y hp coef 1"=w121, "Y lp coef 1"=w120, "Final filter coef"=w25, "PID selector"="PID selector", "X hp coef 1"=w28, "X lp coef 1"=w27, "Final filter coef 2"=w25) -> ("FPGA VI Reference Out"=w122:refnum<k20>, "error out"=w119:errorcluster)
    n149 = in-place {
      in-place-border: [w333] -> w159
      in-place-border: w119 -> [w335]
      n150 = in-place-dvr #6(w165) -> (w334:bool, w332:errorcluster)
      n151 = Compound Arithmetic op=OR(w335, w334, w332) -> (w333:bool)
      n152 = in-place-dvr #6(w333) -> ()  [unwired: 2 out]
    }
    n153 = Or(x="stop", y=w159) -> (x .or. y?=w160:bool)
    n154 = Wait (ms)(milliseconds to wait=u32 33) -> ()  [unwired: 1 out]
  }
  n155 = xnode "Read/Write Control"("FPGA VI Reference In"=w7, "error in"=w8, "stream.request state 2"=3) -> ("FPGA VI Reference Out"=w4:refnum<k20>, "error out"=w6:errorcluster)
  n156 = xnode "Close FPGA VI Reference"("FPGA VI Reference In"=w4, "error in"=w6) -> ("error out"=w15:errorcluster)
  n157 = call <vilib>:"Simple Error Handler.vi"("error in (no error)"=w15) -> ("error out"=→"Error Out":errorcluster)  [unwired: 4 in, 4 out]
